vi "GroveDhtPro.vi"() -> ()   [LabVIEW 2014]
doc: "GrovePi example for using the Grove Temperature & Humidity Sensor Pro (DHT)\n\n(http://www.seeedstudio.com/wiki/Grove_-_Temperature_and_Humidity_Sensor_Pro)"
uses:
  GrovePi/Pin.ctl
  GrovePi/DhtType.ctl
  <vilib>/MakerHub/LINX/Public/Utilities/Open Local.vi
  LinxGrovePi/LinxGrovePi.lvclass
  <vilib>/MakerHub/LINX/LMH-LINX.lvlib
  GrovePi/GrovePi.lvclass
panel:
  in  "DHT Type":T1=1 items=["DHT11", "DHT22", "DHT21", "AM2301"]
  out "Humidity":sgl
  out "Temperature":sgl
  in  "Digital Pin":T2=4 items=["D2"=2, "D3"=3, "D4"=4, "D5"=5, "D6"=6, "D7"=7, "D8"=8, "D9"=9, "A0"=14, "A1"=15, "A2"=16, "A3"=17]
  in  "Stop Button":bool
  out "Error Out":errorcluster
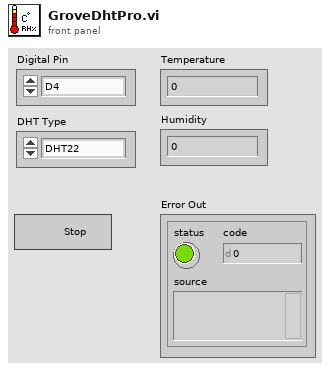
[diagram p1: front panel]
types:
  T1 = typedef "GrovePi.lvclass/DhtType.ctl" = u8
  T2 = typedef "GrovePi.lvclass/Pin.ctl" = u8
  T3 = typedef "LMH-LINX.lvlib/LINX Ref.ctl" = cluster{"IO":T4, "Interface":T5, "LINX Device Config":T6}
  T4 = typedef "LMH-LINX.lvlib/Platform.ctl" = enum16{"Remote", "Local"}
  T5 = typedef "LMH-LINX.lvlib/Interface.ctl" = enum16{"Serial", "TCP"}
  T6 = typedef "LMH-LINX.lvlib/Device.lvlib/LINX Device Config.ctl" = cluster{"Interface":T5, "COM Port":refnum<visa-resource-name>, "TCP Configuration":T7, "Device Family":u8, "Device ID":u8, "Device Name":string, "TCP Ref":refnum<k5>, "Channels":T8}
  T7 = typedef "LMH-LINX.lvlib/Device.lvlib/TCP Config.ctl" = cluster{"IP Address":string, "Port":u16}
  T8 = typedef "LMH-LINX.lvlib/Channels.ctl" = cluster{"DI":u8[], "DO":u8[], "AI":u8[], "AO":u8[], "PWM":u8[], "QE":u8[], "UART":u8[], "I2C 2":u8[], "SPI":u8[], "CAN":u8[], "Servo":u8[], "AI Ref (V)":dbl, "AI Resolution (Bits)":u8, "AO Ref (V)":dbl, "AO Resolution (Bits)":u8}
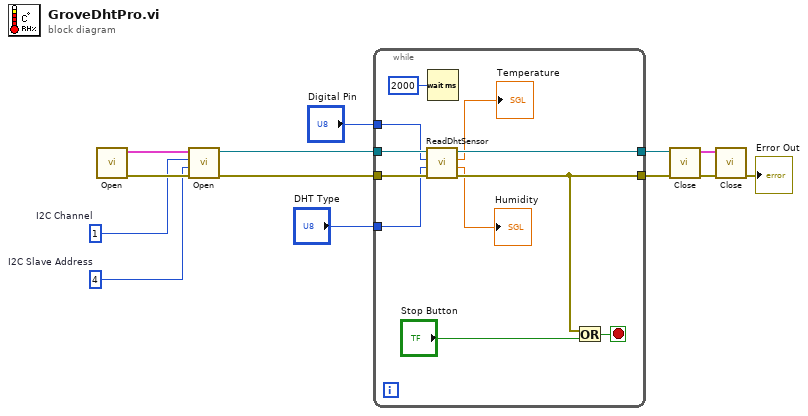
[diagram p0: block diagram]
diagram:
  w9 = u8 4  # I2C Slave Address
  w10 = u8 1  # I2C Channel
  n1 = call-poly <vilib>:"Open.vi"() -> ("Error Out"=w11:errorcluster, "LINX Resource"=w12:T3)  [unwired: 9 in, 1 out]
  n2 = call <vilib>:"Open.vi"("error in (no error)"=w11, "I2C Slave Address (4)"=w9, "I2C Channel (1)"=w10, "LINX Resource"=w12) -> ("error out"=w4:errorcluster, "LINX GrovePi out"=w5:refnum<class "LinxGrovePi.lvclass">)  [unwired: 6 in]
  n3 = while {
    tunnel: [w19] -> w3
    tunnel: [w18] -> w2
    tunnel: w5 -> [w20]
    tunnel: w4 -> [w21]
    tunnel: "Digital Pin" -> [w17]
    tunnel: "DHT Type" -> [w16]
    stop <- w22 stop-if-true
    n4 = call-dynamic "ReadDhtSensor.vi"("error in (no error)"=w21, "DHT Type"=w16, "Digital Pin"=w17, "GrovePi in"=w20) -> ("error out"=w18:errorcluster, "Humidity"=→"Humidity":sgl, "Temperature"=→"Temperature":sgl, "GrovePi out"=w19:refnum<class "LinxGrovePi.lvclass">)  [unwired: 4 in]
    n5 = Wait (ms)(milliseconds to wait=u32 2000) -> ()  [unwired: 1 out]
    n6 = Or(x=w18, y="Stop Button") -> (x .or. y?=w22:bool)
  }
  n7 = call <vilib>:"Close.vi"("error in (no error)"=w2, "LINX GrovePi in"=w3) -> ("error out"=w6:errorcluster, "LINX Resource"=w7:T3)  [unwired: 8 in]
  n8 = call <vilib>:"Close.vi"("Error In"=w6, "LINX Resource"=w7) -> ("Error Out"=→"Error Out":errorcluster)  [unwired: 9 in]
